vi "finishtest.vi"(8 "错误输入（无错误）":errorcluster, 11 "队列输入":refnum<queue>) -> (0 "错误输出":errorcluster, 3 "队列输出":refnum<queue>)   [LabVIEW 2018]
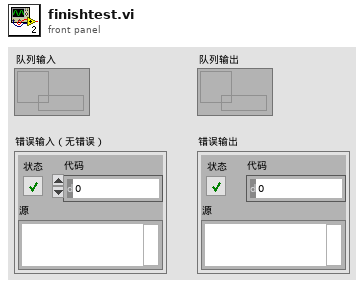
[diagram p1: front panel]
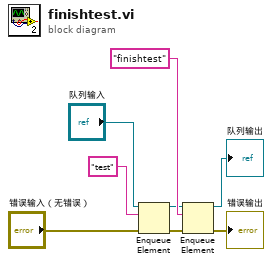
[diagram p0: block diagram]
diagram:
  n1 = Enqueue Element(queue="队列输入", element="test", error in (no error)="错误输入（无错误）") -> (queue out=w3:refnum<queue>, error out=w6:errorcluster)  [unwired: 2 out]
  n2 = Enqueue Element(queue=w3, element="finishtest", error in (no error)=w6) -> (queue out=→"队列输出":refnum<queue>, error out=→"错误输出":errorcluster)  [unwired: 2 out]
